vi "JMsequence.vi"() -> ()   [LabVIEW 2015]
uses:
  <vilib>/Analysis/2dsp.llb/2D Inverse Real FFT.vi
  <vilib>/Analysis/NI_AALPro.lvlib
panel:
  in  "Stop Button":bool
  in  "Tab Control":enum32{"Parameters", "acquisition"}(tab)
  in  "NbX":i32=5
  in  "NbZ":i32=8
  in  "periode T0(us)":dbl=20.0
  in  "N periods":i32=5
  out "Ref duration Target":dbl
  out "Number of frequencies":i32
  out "Number of Frames":i32
  in  "NTrigs":i32=1
  in  "dfx(mm-1)":dbl=0.026
  in  "dfz(mm-1)":dbl=0.0325
  out "inverse FFT":dbl[][](graph)
  out "FFT construct":dbl[][](graph)
  in  "Start Acquire":bool
  in  "index (row)":i32
  in  "disabled index (col)":i32
  in  "fourier value":dbl format="%#_13g"
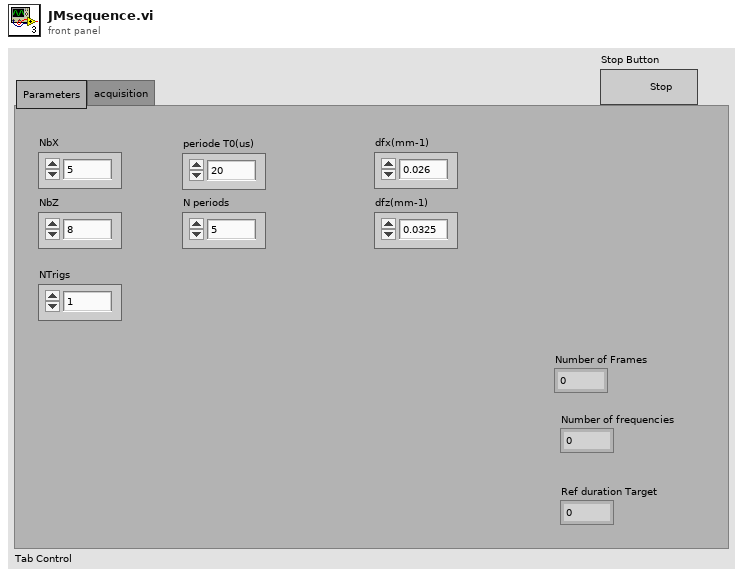
[diagram p1: front panel]
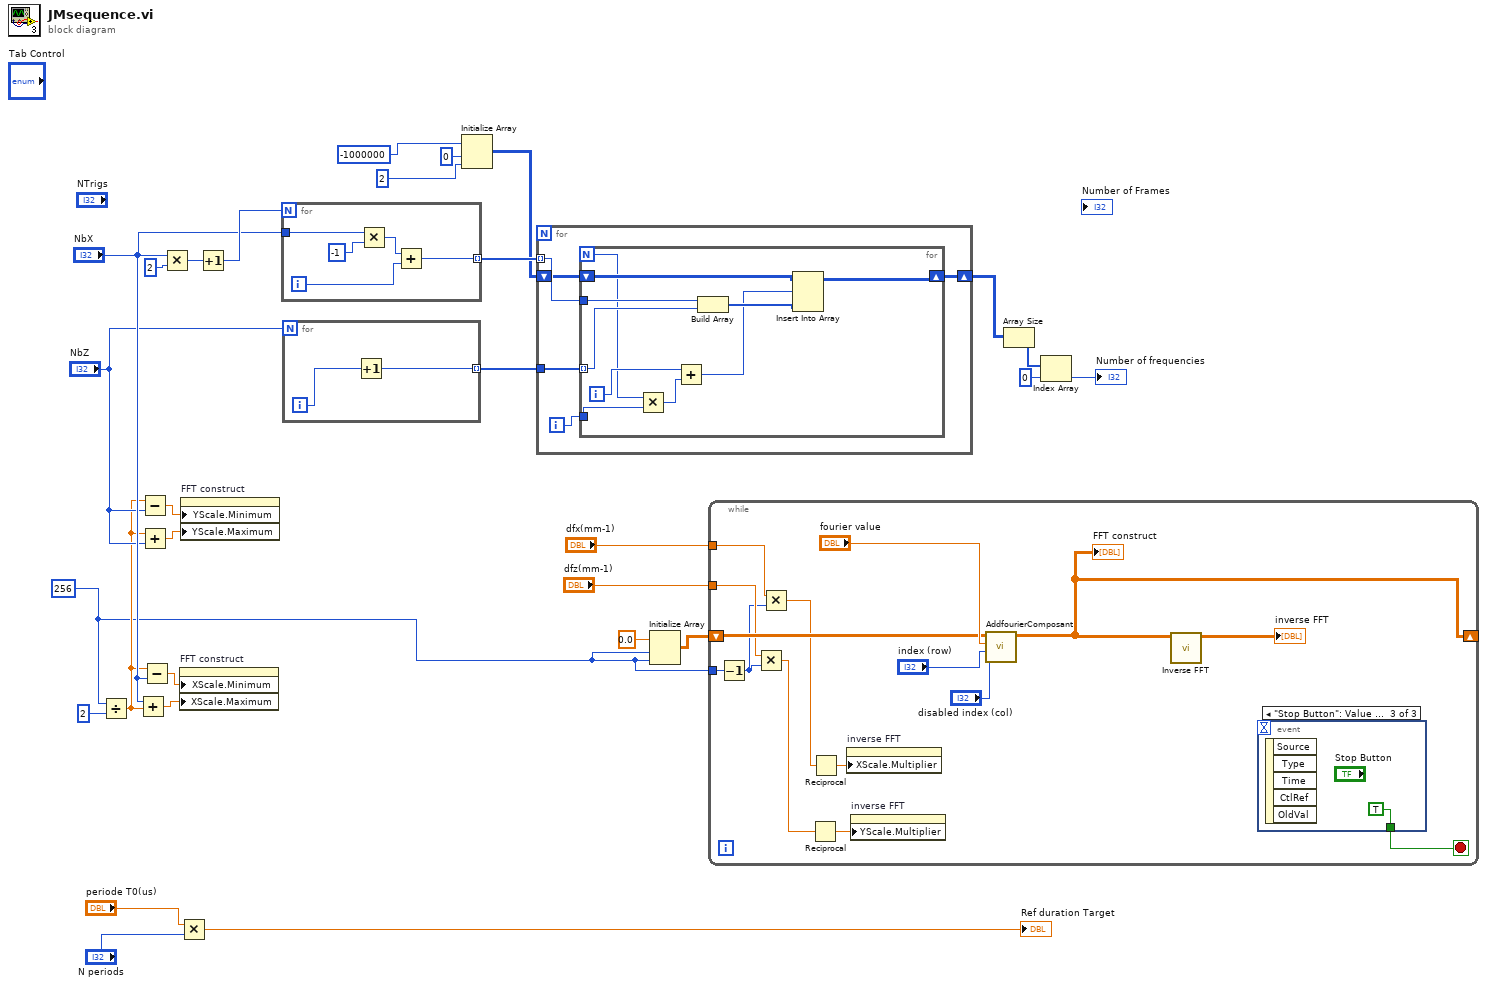
[diagram p0: block diagram]
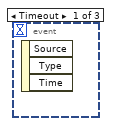
[diagram p2: hidden frame]
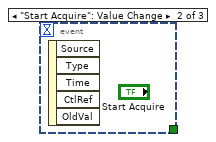
[diagram p3: hidden frame]
diagram:
  w1 = 256 ("dimension size")
  n1 = Divide(x=w1, y=2) -> (x/y=w6:dbl)
  n2 = Add(x="NbX", y=w6) -> (x+y=w8:dbl)
  n3 = Subtract(x=w6, y="NbZ") -> (x-y=w5:dbl)
  n4 = Add(x=w6, y="NbZ") -> (x+y=w4:dbl)
  n5 = Subtract(x=w6, y="NbX") -> (x-y=w9:dbl)
  n6 = Multiply(x="NbX", y=2) -> (x*y=w28:i32)
  n7 = Multiply(x="periode T0(us)", y="N periods") -> (x*y=→"Ref duration Target":dbl)
  n8 = property on="FFT construct" class="IntGraph (strict)"("XScale.Minimum"=w9, "XScale.Maximum"=w8) -> ()  [unwired: 2 in, 2 out]
  n9 = property on="FFT construct" class="IntGraph (strict)"("YScale.Minimum"=w5, "YScale.Maximum"=w4) -> ()  [unwired: 2 in, 2 out]
  n10 = Increment(x=w28) -> (x+1=w25:i32)
  n11 = for {
    N: w25 -> [_]
    tunnel: "NbX" -> [w33]
    tunnel: [w30] -> w23 mode=indexing
    i -> [w31]
    n12 = Multiply(x=w33, y=-1) -> (x*y=w32:i32)
    n13 = Add(x=w32, y=w31) -> (x+y=w30:i32)
  }
  n14 = for {
    N: "NbZ" -> [_]
    tunnel: [w35] -> w22 mode=indexing
    i -> [w36]
    n15 = Increment(x=w36) -> (x+1=w35:i32)
  }
  n16 = Initialize Array(-1000000 ("element"), 0 ("dimension size"), 2 ("dimension size")) -> (w21:i32[][])
  n17 = for {
    tunnel: w23 -> [w40] mode=indexing
    tunnel: w22 -> [w41]
    shift-right: [w38] -> w20
    shift-left: w21 -> [w37]
    i -> [w39]
    n18 = for {
      N -> [w42]
      tunnel: w41 -> [w50] mode=indexing
      tunnel: w40 -> [w51]
      tunnel: w39 -> [w44]
      shift-right: [w46] -> w38
      shift-left: w37 -> [w48]
      i -> [w49]
      n19 = Multiply(x=w42, y=w44) -> (x*y=w43:i32)
      n20 = Add(x=w49, y=w43) -> (x+y=w45:i32)
      n21 = Build Array(w51, w50) -> (w47:i32[])
      n22 = Insert Into Array(array=w48, index (row)=w45, new element=w47) -> (w46:i32[][])  [unwired: 1 in]
    }
  }
  n23 = Initialize Array(0.0 ("r"), w1, w1) -> (w13:dbl[][])
  n24 = while {
    shift-right: [w60] -> _
    shift-left: w13 -> [w61]
    tunnel: "dfx(mm-1)" -> [w56]
    tunnel: "dfz(mm-1)" -> [w58]
    tunnel: w1 -> [w59]
    stop <- w65 stop-if-true
    n25 = Decrement(x=w59) -> (x-1=w57:i32)
    n26 = Multiply(x=w58, y=w57) -> (x*y=w53:dbl)
    n27 = Multiply(x=w56, y=w57) -> (x*y=w54:dbl)
    n28 = Reciprocal(x=w53) -> (1/x=w52:dbl)
    n29 = Reciprocal(x=w54) -> (1/x=w55:dbl)
    n30 = property on="inverse FFT" class="IntGraph (strict)"("XScale.Multiplier"=w55) -> ()  [unwired: 2 in, 2 out]
    n31 = property on="inverse FFT" class="IntGraph (strict)"("YScale.Multiplier"=w52) -> ()  [unwired: 2 in, 2 out]
    n32 = call "AddfourierComposant.vi"("disabled index (col)"="disabled index (col)", "index (row)"="index (row)", 10:"fourier value", "FFT matrix"=w61) -> ("output array"=w60:dbl[][])  [unwired: 7 in]
    "FFT construct" <- w60
    n33 = call-poly <vilib>:"Inverse FFT.vi"("FFT {X}"=w60) -> ("X"=→"inverse FFT":dbl[][])  [unwired: 9 in, 1 out]
    n34 = event shown="[2] \"Stop Button\": Value Change" {
      selector: _ -> [_ _ _]
      dyn-events: _ -> [_ _ _]
      timeout: _ -> [_ _ _]
      tunnel: [_ _ TRUE] -> w65
      event Timeout {
        n35 = event-data() -> ()  [unwired: 1 in, 3 out]
      }
      event "Start Acquire": Value Change {
        n36 = event-data() -> ()  [unwired: 1 in, 5 out]
      }
      event "Stop Button": Value Change {
        n37 = event-data() -> ()  [unwired: 1 in, 5 out]
      }
    }
  }
  n38 = Array Size(array=w20) -> (size(s)=w19:i32[])
  n39 = Index Array(array=w19, index=0) -> (element=→"Number of frequencies":i32)
